vi "GUI_Initialize.vi"(4 "error in (no error)":errorcluster) -> (0 "error out":errorcluster, 1 "Canceled?":bool, 2 "Initialize Out":T1)   [LabVIEW 2015]
doc: "A GUI that allows the user to chose the systems that should be initialized."
uses:
  Systems/TCS_Link/TCSLINK_global.vi
panel:
  in  "Listbox":i32(listbox)=7
  in  "None":bool
  in  "All":bool
  in  "Home Selectedl":bool
  # "Double click to change a system's status"
  # "Assure that each componentis clear of interference before homing.  A homing sequence will be initiated for each selected system. You will not have control of uninitialized systems."
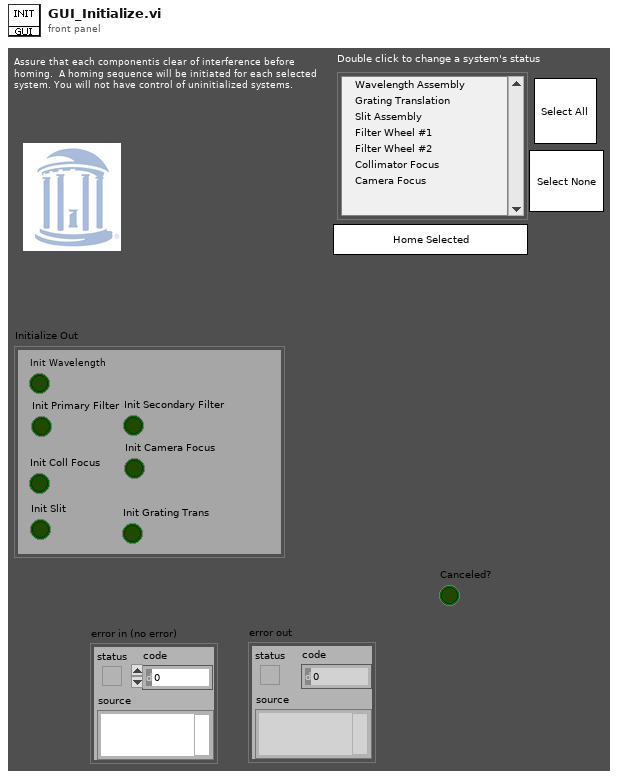
[diagram p1: front panel]
types:
  T1 = cluster{"Init Primary Filter":bool, "Init Secondary Filter":bool, "Init Coll Focus":bool, "Init Camera Focus":bool, "Init Slit":bool, "Init Grating Trans":bool, "Init Wavelength":bool}
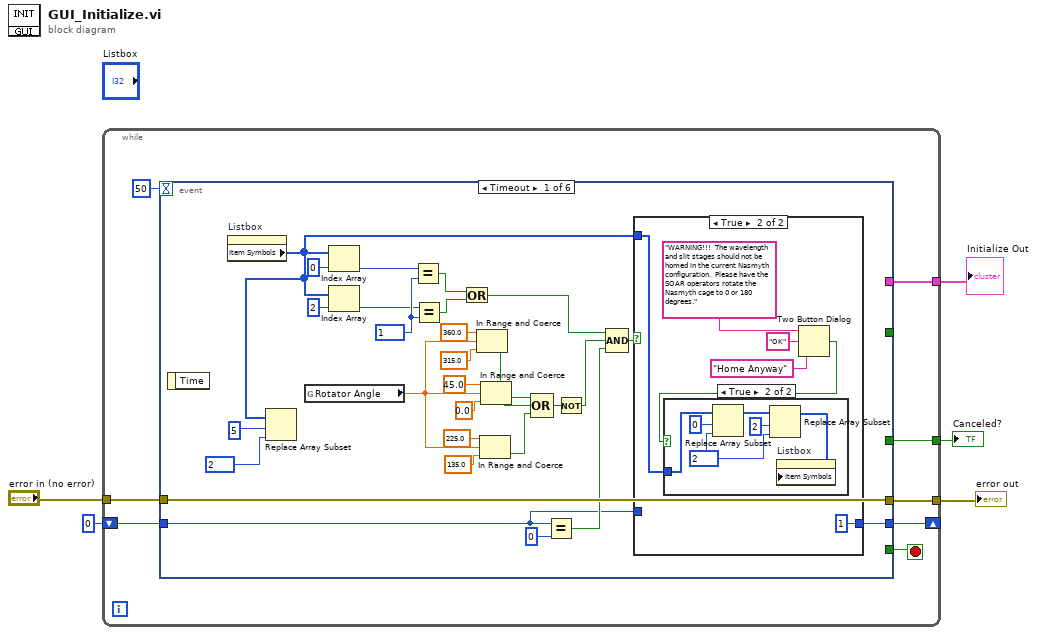
[diagram p0: block diagram]
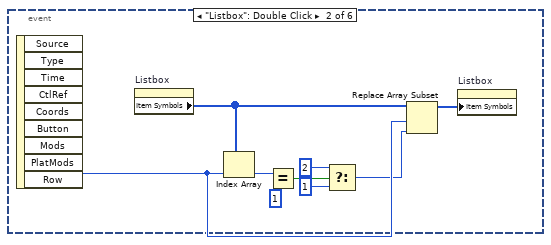
[diagram p4: hidden frame]
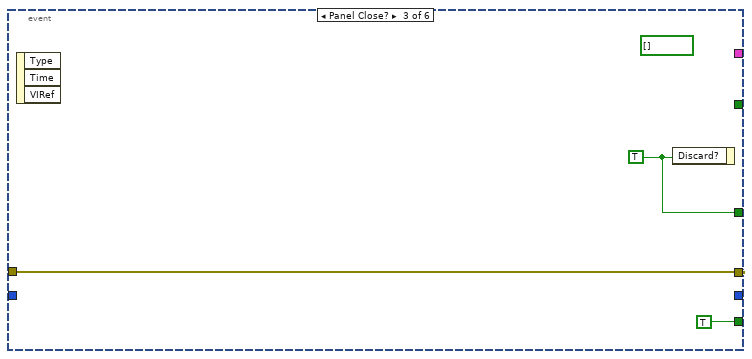
[diagram p5: hidden frame]
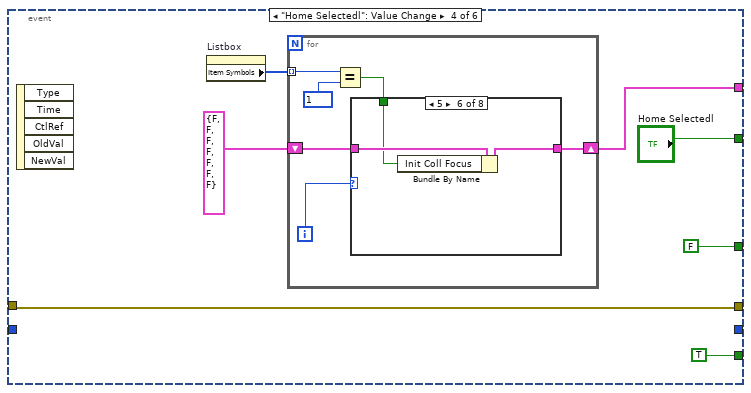
[diagram p6: hidden frame]
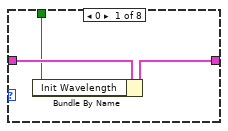
[diagram p7: hidden frame]
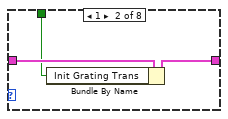
[diagram p8: hidden frame]
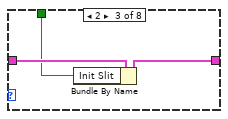
[diagram p9: hidden frame]
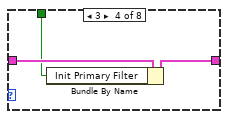
[diagram p10: hidden frame]
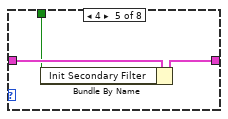
[diagram p11: hidden frame]
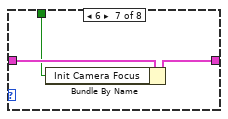
[diagram p12: hidden frame]
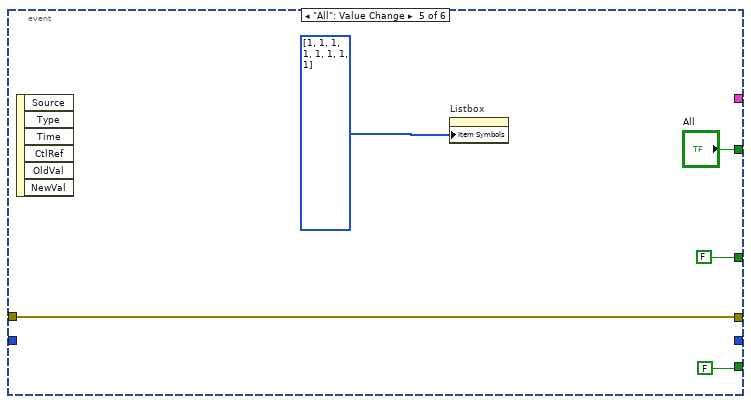
[diagram p14: hidden frame]
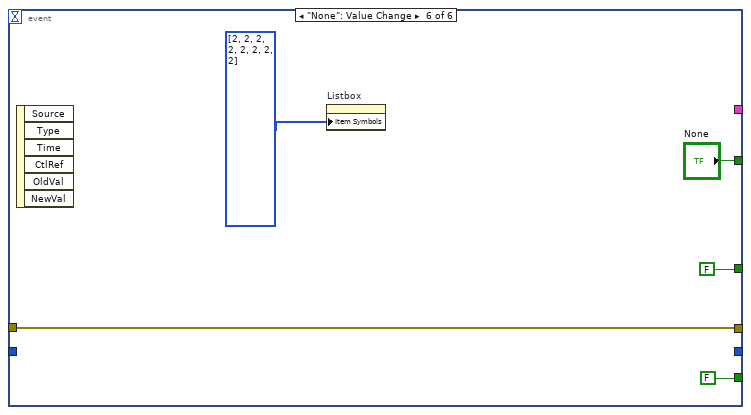
[diagram p15: hidden frame]
diagram:
  n1 = while {
    tunnel: "error in (no error)" -> [w13]
    tunnel: [w12] -> w4
    tunnel: [w11] -> w3
    tunnel: [w9] -> w2
    shift-right: [w6] -> _
    shift-left: 0 ("index") -> [w7]
    stop <- w10 stop-if-true
    n2 = event shown="[0] Timeout" {
      selector: _ -> [_ _ _ _ _ _]
      dyn-events: _ -> [_ _ _ _ _ _]
      timeout: 50 -> [_ _ _ _ _ _]
      tunnel: [w42 _ w67 w72 w106 w111] -> w12
      tunnel: w13 -> [w42 _ w67 w72 w106 w111]
      tunnel: [_ _ _ "Home Selectedl" "All" "None"] -> _
      tunnel: [_ _ w65 FALSE ("Canceled?") FALSE FALSE] -> w11
      tunnel: [_ _ TRUE TRUE FALSE FALSE] -> w10
      tunnel: [_ _ _ w69 _ _] -> w9
      tunnel: w7 -> [w17 _ _ _ _ _]
      tunnel: [w18 _ _ _ _ _] -> w6
      event Timeout {
        w39 = 1
        n3 = event-data() -> ()  [unwired: 1 in, 1 out]
        n4 = property on="Listbox" class="LstBox (strict)"() -> ("Item Symbols"=w16:i32[])  [unwired: 2 in, 2 out]
        n5 = Replace Array Subset(array=w16, new element=2, index=5) -> ()  [unwired: 1 out]
        n6 = global read "TCSLINK_global.vi" "Rotator Angle"() -> (w24:dbl)
        n7 = Index Array(array=w16, index=0) -> (element=w37:i32)
        n8 = Index Array(array=w16, index=2) -> (element=w38:i32)
        n9 = Equal?(x=w37, y=w39) -> (x = y?=w36:bool)
        n10 = Equal?(x=w38, y=w39) -> (x = y?=w35:bool)
        n11 = Or(x=w36, y=w35) -> (x .or. y?=w23:bool)
        n12 = In Range and Coerce(upper limit=360.0, x=w24, lower limit=315.0) -> (In Range?=w28:bool)  [unwired: 1 out]
        n13 = In Range and Coerce(upper limit=225.0, x=w24, lower limit=135.0) -> (In Range?=w26:bool)  [unwired: 1 out]
        n14 = In Range and Coerce(upper limit=45.0, x=w24, lower limit=0.0) -> (In Range?=w27:bool)  [unwired: 1 out]
        n15 = Compound Arithmetic op=OR(w28, w27, w26) -> (w25:bool)
        n16 = Equal?(x=w17, y=0 ("index")) -> (x = y?=w19:bool)
        n17 = Not(x=w25) -> (.not. x?=w22:bool)
        n18 = Compound Arithmetic op=AND(w23, w22, w19) -> (w21:bool)
        n19 = case shown="True" w21 {
          tunnel: w16 -> [_ w49]
          tunnel: [w43 1 ("index")] -> w18
          tunnel: w17 -> [w43 _]
          frame False {
          }
          frame True {
            n20 = Two Button Dialog(message="WARNING!!!  The wavelength and slit stages should not be homed in the current Nasmyth configuration.  Please have the SOAR operators rotate the Nasmyth cage to 0 or 180 degrees.", 1:"Home Anyway" ("F button name (\"Cancel\")"), 2:"OK" ("T button name (\"OK\")")) -> (T button?=w45:bool)
            n21 = case shown="True" w45 {
              tunnel: w49 -> [_ w53]
              frame False {
              }
              frame True {
                w51 = 2
                n22 = Replace Array Subset(array=w53, new element=w51, index=0) -> (w52:i32[])
                n23 = Replace Array Subset(array=w52, new element=w51, index=2) -> (w50:i32[])
                n24 = property on="Listbox" class="LstBox (strict)"("Item Symbols"=w50) -> ()  [unwired: 2 in, 2 out]
              }
            }
          }
        }
      }
      event "Listbox": Double Click {
        n25 = event-data() -> ("Row"=w58:i32)  [unwired: 1 in, 8 out]
        n26 = property on="Listbox" class="LstBox (strict)"() -> ("Item Symbols"=w59:i32[])  [unwired: 2 in, 2 out]
        n27 = Index Array(array=w59, index=w58) -> (element=w64:i32)
        n28 = Equal?(x=w64, y=1) -> (x = y?=w62:bool)
        n29 = Select(t=2, s=w62, f=1) -> (s? t:f=w57:i32)
        n30 = Replace Array Subset(array=w59, new element=w57, index=w58) -> (w56:i32[])
        n31 = property on="Listbox" class="LstBox (strict)"("Item Symbols"=w56) -> ()  [unwired: 2 in, 2 out]
      }
      event Panel Close? {
        (unwired) bool[] [] ("Initialize")
        w65 = TRUE ("Canceled?")
        n32 = event-data() -> ()  [unwired: 1 in, 3 out]
        n33 = event-data("Discard?"=w65) -> ()  [unwired: 1 in, 1 out]
      }
      event "Home Selectedl": Value Change {
        n34 = event-data() -> ()  [unwired: 1 in, 5 out]
        n35 = property on="Listbox" class="LstBox (strict)"() -> ("Item Symbols"=w71:i32[])  [unwired: 2 in, 2 out]
        n36 = for {
          tunnel: w71 -> [w80] mode=indexing
          shift-right: [w77] -> w69
          shift-left: T1 {"Init Primary Filter"=FALSE, "Init Secondary Filter"=FALSE, "Init Coll Focus"=FALSE, "Init Camera Focus"=FALSE, "Init Slit"=FALSE, "Init Grating Trans"=FALSE, "Init Wavelength"=FALSE} ("Initialize Out") -> [w78]
          i -> [w79]
          n37 = Equal?(x=w80, y=1) -> (x = y?=w76:bool)
          n38 = case shown="5" w79 {
            tunnel: w78 -> [w83 w86 w89 w92 w95 w98 w101 w102]
            tunnel: [w82 w85 w88 w91 w94 w97 w100 w102] -> w77
            tunnel: w76 -> [w81 w84 w87 w90 w93 w96 w99 _]
            frame 0 {
              n39 = Bundle By Name(cluster=w83, "Init Wavelength"=w81) -> (w82:T1)
            }
            frame 1 {
              n40 = Bundle By Name(cluster=w86, "Init Grating Trans"=w84) -> (w85:T1)
            }
            frame 2 {
              n41 = Bundle By Name(cluster=w89, "Init Slit"=w87) -> (w88:T1)
            }
            frame 3 {
              n42 = Bundle By Name(cluster=w92, "Init Primary Filter"=w90) -> (w91:T1)
            }
            frame 4 {
              n43 = Bundle By Name(cluster=w95, "Init Secondary Filter"=w93) -> (w94:T1)
            }
            frame 5 {
              n44 = Bundle By Name(cluster=w98, "Init Coll Focus"=w96) -> (w97:T1)
            }
            frame 6 {
              n45 = Bundle By Name(cluster=w101, "Init Camera Focus"=w99) -> (w100:T1)
            }
            frame 7, Default {
            }
          }
        }
      }
      event "All": Value Change {
        n46 = event-data() -> ()  [unwired: 1 in, 6 out]
        n47 = property on="Listbox" class="LstBox (strict)"("Item Symbols"=i32[] [1, 1, 1, 1, 1, 1, 1, 1]) -> ()  [unwired: 2 in, 2 out]
      }
      event "None": Value Change {
        n48 = event-data() -> ()  [unwired: 1 in, 6 out]
        n49 = property on="Listbox" class="LstBox (strict)"("Item Symbols"=i32[] [2, 2, 2, 2, 2, 2, 2, 2]) -> ()  [unwired: 2 in, 2 out]
      }
    }
  }
  "error out" <- w4
  "Canceled?" <- w3
  "Initialize Out" <- w2
